vi "Write Loaded test recipe.vi"(7 "Send any changes now? (F)":bool, 8 "error in (no error)":errorcluster, 10 "Loaded test recipe":refnum<class "Test Recipe.lvclass">, 11 "Fiber Auto Collimation state data in":refnum<class "Fiber Auto Collimation state data.lvclass">) -> (0 "error out":errorcluster, 3 "Fiber Auto Collimation state data out":refnum<class "Fiber Auto Collimation state data.lvclass">)   [LabVIEW 2018, in "Fiber Auto Collimation state data.lvclass"]
uses:
  Fiber Auto Collimation state data.lvclass
  <userlib>/Recipe/Test Recipe classes/Test Recipe.lvclass
  Fiber Auto Collimation state data.lvclass/Fiber Auto Collimation state data.ctl
  Tracked state data.ctl
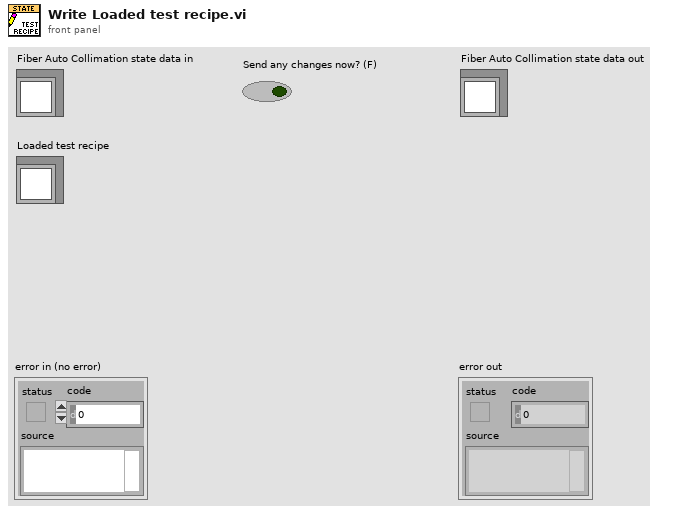
[diagram p1: front panel]
types:
  T1 = typedef "Fiber Auto Collimation state data.lvclass/Tracked state data.ctl" = enum16{"No update", "Permission level", "Username", "Test running", "DUT Serial", "Test status", "MOM Lot", "Loaded test recipe", "Model case running", "Station status", "BV data", "Defect Identify data", "Axis Position data", "Fiber Ass PN", "Operator", "RunTime", "VBAI", "Steps Cycle Time"}
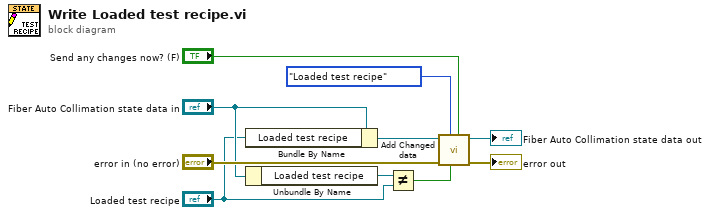
[diagram p0: block diagram]
diagram:
  n1 = Bundle By Name(cluster="Fiber Auto Collimation state data in", "Loaded test recipe"="Loaded test recipe") -> (w8:refnum<class "Fiber Auto Collimation state data.lvclass">)
  n2 = Unbundle By Name("Fiber Auto Collimation state data in") -> ("Loaded test recipe"=w4:refnum<class "Test Recipe.lvclass">)
  n3 = Not Equal?(x=w4, y="Loaded test recipe") -> (x != y?=w5:bool)
  n4 = call "Add Changed data.vi"("Send any changes now? (F)"="Send any changes now? (F)", "Data changed?"=w5, "Data type"=Tracked_state_data."Loaded test recipe", "error in (no error)"="error in (no error)", "Fiber Auto Collimation state data in"=w8) -> ("error out"=→"error out":errorcluster, "Fiber Auto Collimation state data out"=→"Fiber Auto Collimation state data out":refnum<class "Fiber Auto Collimation state data.lvclass">)  [unwired: 5 in]
